vi "p1.vi"() -> ()   [LabVIEW 2021, in "d23.lvlib"]
uses:
  d23.lvlib
  AOC/AOC.lvlib
panel:
  in  "Example":string=".....\n..##.\n..#..\n.....\n..##.\n....."
  in  "Example":bool=TRUE
  out "Answer":i64
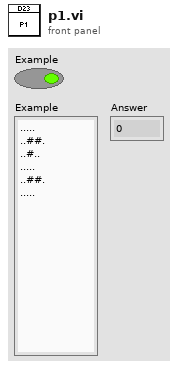
[diagram p1: front panel]
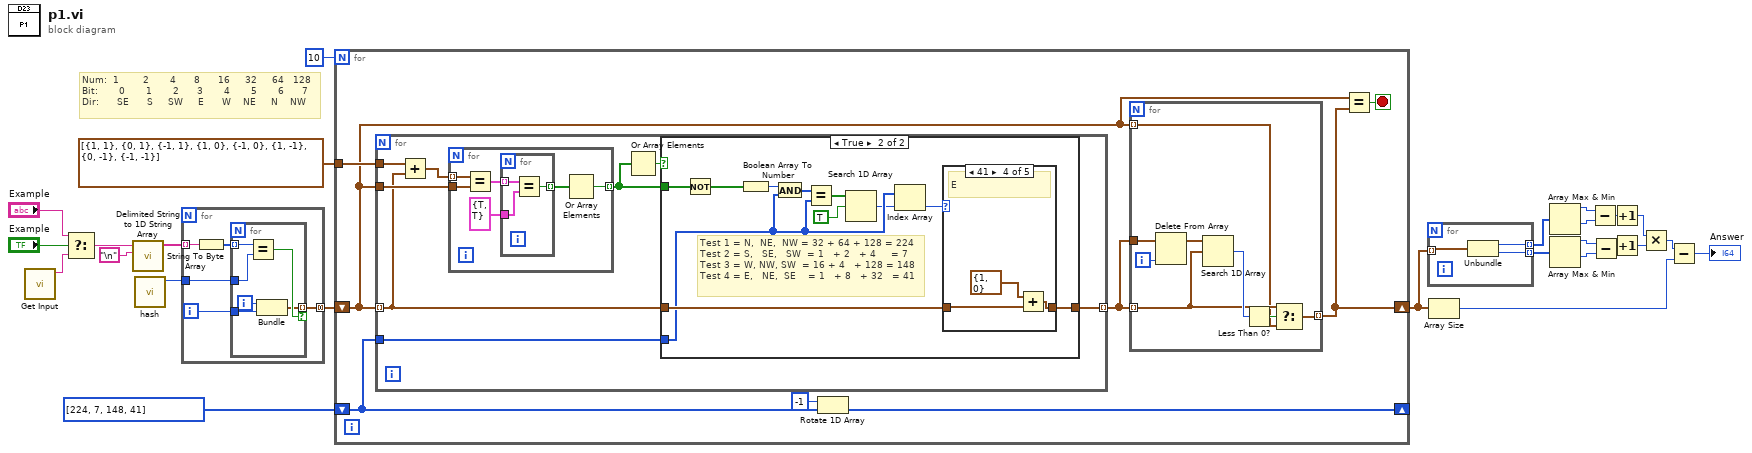
[diagram p0: block diagram]
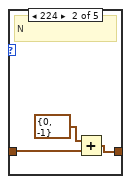
[diagram p4: hidden frame]
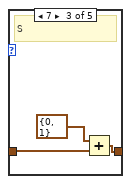
[diagram p5: hidden frame]
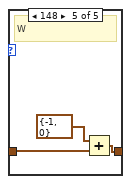
[diagram p6: hidden frame]
diagram:
  # "Num:  1        2       4      8      16     32     64   128\nBit:       0       1       2      3       4       5       6      7\nDir:      SE      S     SW     E      W    NE     N    NW"
  n1 = call "Get Input.vi"() -> ("Input"=w25:string)  [unwired: 11 in]
  n2 = Select(t="Example", s="Example", f=w25) -> (s? t:f=w24:string)
  n3 = call <vilib>:"Delimited String to 1D String Array.vi"("delimiter"="\n", "delimited string"=w24) -> ("string array"=w20:string[])  [unwired: 9 in]
  n4 = call "hash.vi"() -> ("#"=w19:u8)  [unwired: 11 in]
  n5 = for {
    tunnel: w20 -> [w30] mode=indexing
    tunnel: w19 -> [w28]
    tunnel: [w27] -> w17 mode=concatenating
    i -> [w26]
    n6 = String To Byte Array(string=w30) -> (unsigned byte array=w29:u8[])
    n7 = for {
      tunnel: w29 -> [w36] mode=indexing
      tunnel: w28 -> [w35]
      tunnel: [w33] -> w27 mode=indexing if=w34
      tunnel: w26 -> [w32]
      i -> [w31]
      n8 = Equal?(x=w36, y=w35) -> (x = y?=w34:bool)
      n9 = Bundle(w31, w32) -> (w33:cluster{i32, i32})  [unwired: 1 in]
    }
  }
  n10 = for {
    N: 10 -> [_]
    shift-right: [w37] -> w5
    shift-left: w17 -> [w39]
    tunnel: cluster{i32, i32}[] [{1, 1}, {0, 1}, {-1, 1}, {1, 0}, {-1, 0}, {1, -1}, {0, -1}, {-1, -1}] -> [w44]
    shift-right: [w41] -> _
    shift-left: u8[] [224, 7, 148, 41] ("number") -> [w42]
    stop <- w38 stop-if-true
    n11 = for {
      tunnel: w39 -> [w56] mode=indexing
      tunnel: w39 -> [w59]
      tunnel: w44 -> [w57]
      tunnel: [w54] -> w43 mode=indexing
      tunnel: w42 -> [w53]
      n12 = Add(x=w57, y=w56) -> (x+y=w60:cluster{i32, i32}[])
      n13 = for {
        tunnel: w60 -> [w66] mode=indexing
        tunnel: w59 -> [w65]
        tunnel: [w61] -> w55 mode=indexing
        n14 = Equal?(x=w66, y=w65) -> (x = y?=w64:cluster{bool, bool}[])
        n15 = for {
          tunnel: w64 -> [w69] mode=indexing
          tunnel: cluster{bool, bool} {TRUE, TRUE} ("y") -> [w68]
          tunnel: [w67] -> w62 mode=indexing
          n16 = Equal?(x=w69, y=w68) -> (x = y?=w67:bool)
        }
        n17 = Or Array Elements(Boolean array=w62) -> (logical OR=w61:bool)
      }
      n18 = Or Array Elements(Boolean array=w55) -> (logical OR=w58:bool)
      n19 = case shown="True" w58 {
        tunnel: w56 -> [w70 w81]
        tunnel: [w70 w78] -> w54
        tunnel: w55 -> [_ w79]
        tunnel: w53 -> [_ w73]
        frame False {
        }
        frame True {
          # "Test 1 = N,  NE,  NW = 32 + 64 + 128 = 224\nTest 2 = S,   SE,   SW  = 1   + 2   + 4     = 7\nTest 3 = W, NW, SW  = 16 + 4   + 128 = 148\nTest 4 = E,   NE,  SE    = 1   + 8   + 32   = 41"
          n20 = Not(x=w79) -> (.not. x?=w77:bool[])
          n21 = Boolean Array To Number(Boolean array=w77) -> (number=w80:u8)
          n22 = And(x=w80, y=w73) -> (x .and. y?=w76:u8[])
          n23 = Equal?(x=w76, y=w73) -> (x = y?=w75:bool[])
          n24 = Search 1D Array(1D array=w75, element=TRUE) -> (index of element=w72:i32)  [unwired: 1 in]
          n25 = Index Array(array=w73, index=w72) -> (element=w71:u8)
          n26 = case shown="41" w71 {
            tunnel: w81 -> [w82 w84 w87 w90 w93]
            tunnel: [w82 w83 w86 w89 w92] -> w78
            frame Default {
              # "Can't Move"
            }
            frame 224 {
              # "N"
              n27 = Add(x=cluster{i32, i32} {0, -1}, y=w84) -> (x+y=w83:cluster{i32, i32})
            }
            frame 7 {
              # "S"
              n28 = Add(x=cluster{i32, i32} {0, 1}, y=w87) -> (x+y=w86:cluster{i32, i32})
            }
            frame 41 {
              # "E"
              n29 = Add(x=cluster{i32, i32} {1, 0}, y=w90) -> (x+y=w89:cluster{i32, i32})
            }
            frame 148 {
              # "W"
              n30 = Add(x=cluster{i32, i32} {-1, 0}, y=w93) -> (x+y=w92:cluster{i32, i32})
            }
          }
        }
      }
    }
    n31 = Rotate 1D Array(1:w42, 2:-1 ("n")) -> (0:w41:u8[])
    n32 = for {
      tunnel: w43 -> [w47] mode=indexing
      tunnel: w39 -> [w46] mode=indexing
      tunnel: w43 -> [w52]
      tunnel: [w45] -> w37 mode=indexing
      i -> [w51]
      n33 = Delete From Array(array=w52, index=w51) -> (array with subset deleted=w50:cluster{i32, i32}[])  [unwired: 1 in, 1 out]
      n34 = Search 1D Array(1D array=w50, element=w47) -> (index of element=w49:i32)  [unwired: 1 in]
      n35 = Less Than 0?(x=w49) -> (x < 0?=w48:bool)
      n36 = Select(t=w47, s=w48, f=w46) -> (s? t:f=w45:cluster{i32, i32})
    }
    n37 = Equal?(x=w39, y=w37) -> (x = y?=w38:bool)
  }
  n38 = for {
    tunnel: w5 -> [w97] mode=indexing
    tunnel: [w96] -> w6 mode=indexing
    tunnel: [w95] -> w7 mode=indexing
    n39 = Unbundle(w97) -> (w96:i32, w95:i32)
  }
  n40 = Array Size(array=w5) -> (size(s)=w11:i32)
  n41 = Array Max & Min(array=w6) -> (max value=w4:i32, min value=w1:i32)  [unwired: 2 out]
  n42 = Array Max & Min(array=w7) -> (max value=w3:i32, min value=w2:i32)  [unwired: 2 out]
  n43 = Subtract(x=w4, y=w1) -> (x-y=w13:i32)
  n44 = Subtract(x=w3, y=w2) -> (x-y=w14:i32)
  n45 = Increment(x=w13) -> (x+1=w9:i32)
  n46 = Increment(x=w14) -> (x+1=w8:i32)
  n47 = Multiply(x=w9, y=w8) -> (x*y=w12:i32)
  n48 = Subtract(x=w12, y=w11) -> (x-y=→"Answer":i32)
